vi "Simple VFH Evaluate Current Gap.vi"(5 "total sample size":i32, 6 "size of best gap so far":i32, 7 "size of gap":i32, 8 "offset of best gap so far":i32, 9 "offset of end of gap":i32) -> (0 "new winner?":bool, 1 "winning score":dbl, 2 "size of best gap so far":i32, 3 "offset of best gap so far":i32)   [LabVIEW 2017, in "NI_Robotics_Simple Vector Field Histogram.lvlib"]
uses:
  <vilib>/robotics/Obstacle Avoidance/Simple Vector Field Histogram/NI_Robotics_Simple Vector Field Histogram.lvlib
  <vilib>/gmath/statdist.llb/Continuous PDF.vi
  <vilib>/gmath/statdist.llb/Normal PDF.vi
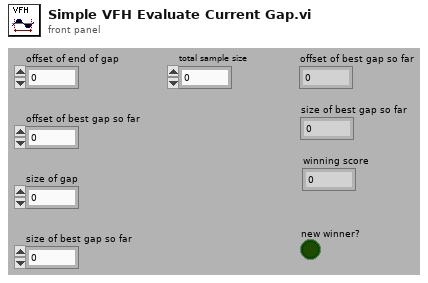
[diagram p1: front panel]
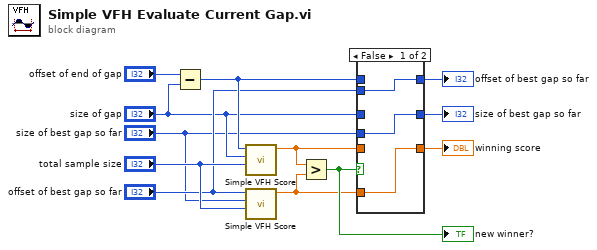
[diagram p0: block diagram]
diagram:
  n1 = Subtract(x="offset of end of gap", y="size of gap") -> (x-y=w10:i32)
  n2 = call <vilib>:"Simple VFH Score.vi"("total sample size"="total sample size", "size of best gap so far"="size of gap", "offset of best gap so far"=w10) -> ("score"=w4:dbl)  [unwired: 8 in]
  n3 = call <vilib>:"Simple VFH Score.vi"("total sample size"="total sample size", "size of best gap so far"="size of best gap so far", "offset of best gap so far"="offset of best gap so far") -> ("score"=w1:dbl)  [unwired: 8 in]
  n4 = Greater?(x=w4, y=w1) -> (0:w2:bool)
  "new winner?" <- w2
  n5 = case shown="False" w2 {
    tunnel: w10 -> [_ w18]
    tunnel: [w15 w18] -> w9
    tunnel: "offset of best gap so far" -> [w15 _]
    tunnel: "size of gap" -> [_ w17]
    tunnel: [w14 w17] -> w6
    tunnel: "size of best gap so far" -> [w14 _]
    tunnel: w4 -> [_ w16]
    tunnel: [w13 w16] -> w3
    tunnel: w1 -> [w13 _]
    frame False {
    }
    frame True {
    }
  }
  "offset of best gap so far" <- w9
  "size of best gap so far" <- w6
  "winning score" <- w3
